vi "APU Page.vi"(8 "error in (no error)":errorcluster, 11 "Node Ptr":T1 format="%.0x") -> (0 "error out":errorcluster)   [LabVIEW 2015, in "Engine Simulation Toolkit System Explorer.lvlib"]
uses:
  Engine Simulation Toolkit System Explorer.lvlib
  <vilib>/NI Veristand/Custom Device API/Custom Device Item Ref.ctl
  Shared/Properties.vi
  <vilib>/NI Veristand/Custom Device API/Get Item Property (U16).vi
  <vilib>/NI Veristand/Custom Device API/Get Item Property (Double).vi
  <vilib>/NI Veristand/Custom Device API/Get Item Property (String).vi
  <vilib>/NI Veristand/Custom Device API/Get Item Property (Boolean).vi
  Shared/Constants and GUIDs.vi
  <vilib>/NI Veristand/Custom Device Tools/Custom Device Utility Library/NI VeriStand - Search for Item by Name.vi
  <vilib>/NI Veristand/Custom Device API/Set Item Property (Double).vi
  <vilib>/NI Veristand/Custom Device API/Set Item Property (Boolean).vi
  <vilib>/NI Veristand/Custom Device API/Custom Device API.lvlib
  Shared/Engine Simulation Toolkit Shared.lvlib
  <vilib>/NI Veristand/Custom Device Tools/Custom Device Utility Library/Custom Device Utility Library.lvlib
panel:
  in  "des speed":dbl caption="Start speed (RPM)"
  in  "Start angle (degrees)":dbl
  in  "des accel":dbl caption="Acceleration (RPM/sec)" min=0.0 format="%#_p"
  in  "Acceleration":bool
  out "Name in bitfile":string
  in  "Header":cluster{"Section Name":string}={"Section Name"="APU Settings"}
  in  "Description":string
  in  "Name":string
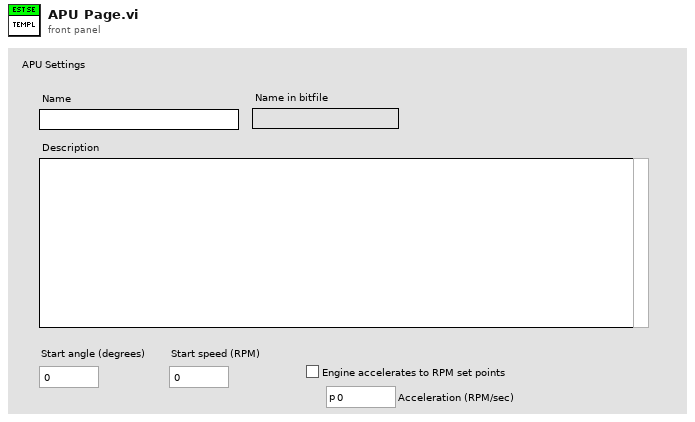
[diagram p1: front panel]
types:
  T1 = typedef "Custom Device API.lvlib/Custom Device Item Ref.ctl" = u64
  T2 = enum8{"Enabled", "Disabled", "Disabled and Grayed Out"}
  T3 = typedef "Engine Simulation Toolkit Shared.lvlib/Channel.ctl" = cluster{"Name":string, "Units":string, "Default":dbl, "Description":string}
  T4 = typedef "Custom Device API.lvlib/Custom Device Channel.ctl" = cluster{"Type":T5, "Units":string, "Default Value":dbl, "Faultable":bool, "Scalable":bool}
  T5 = typedef "Custom Device API.lvlib/Custom Device Channel Type.ctl" = enum16{"Input", "Output"}
  T6 = typedef "Custom Device API.lvlib/Custom Device Item Info.ctl" = cluster{"Name":string, "Is Channel":bool, "GUID":string, "Is Waveform":bool}
  T7 = typedef "Custom Device API.lvlib/Custom Device Commands.ctl" = enum16{"Default", "Item renamed", "Shutdown", "Dynamic button pressed"}
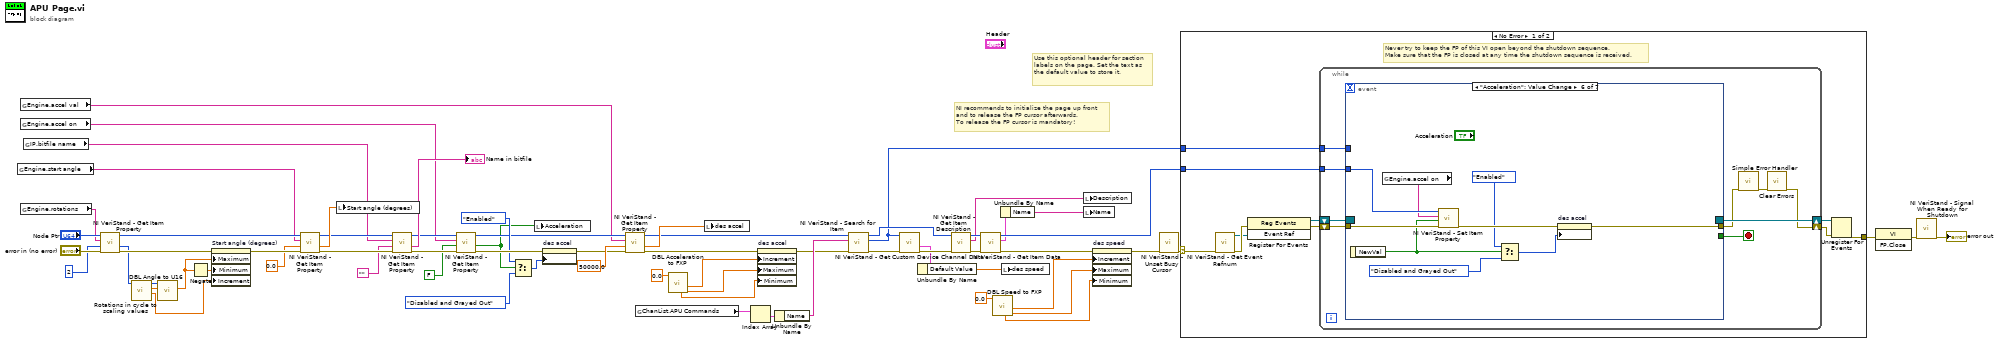
[diagram p0: block diagram]
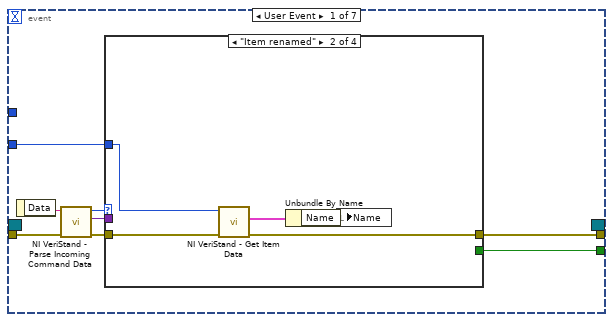
[diagram p2: hidden frame]
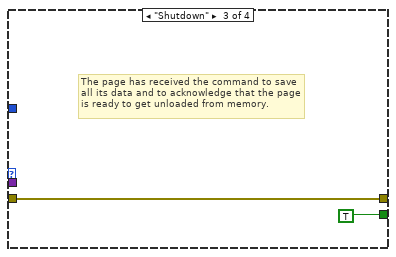
[diagram p4: hidden frame]
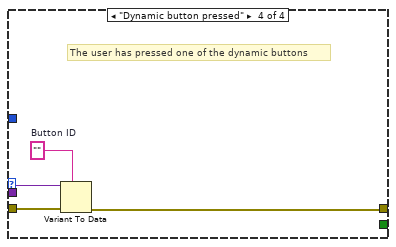
[diagram p5: hidden frame]
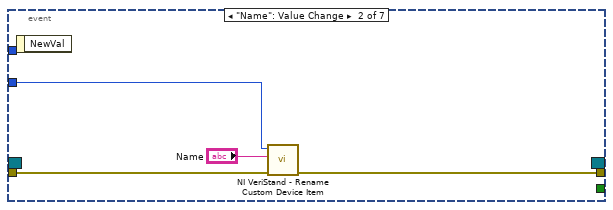
[diagram p6: hidden frame]
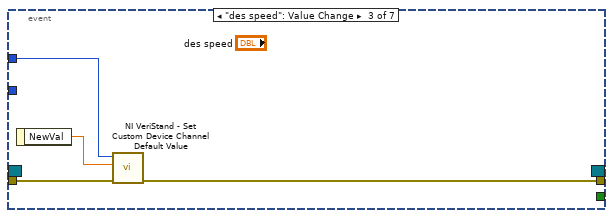
[diagram p7: hidden frame]
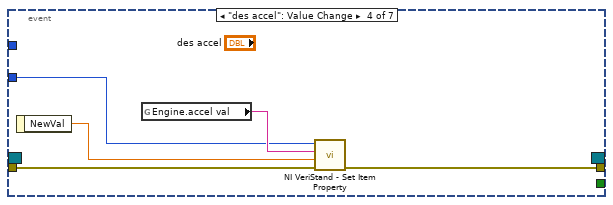
[diagram p8: hidden frame]
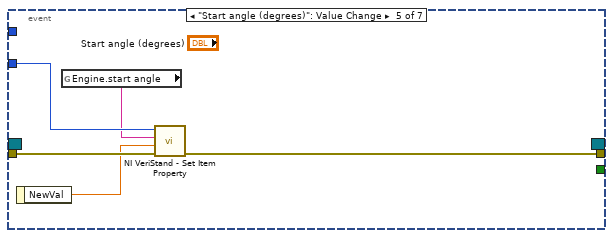
[diagram p9: hidden frame]
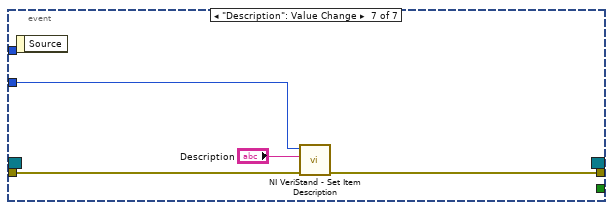
[diagram p10: hidden frame]
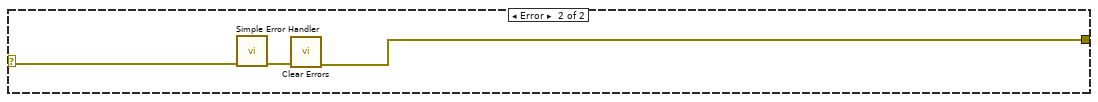
[diagram p11: hidden frame]
diagram:
  # "Use this optional header for section labels on the page. Set the text as the default value to store it."
  # "NI recommends to initialize the page up front\nand to release the FP cursor afterwards.\nTo release the FP cursor is mandatory!"
  n1 = global read "Properties.vi" "Engine.start angle"() -> (w50:string)
  n2 = global read "Properties.vi" "Engine.rotations"() -> (w54:string)
  n3 = global read "Properties.vi" "Engine.accel val"() -> (w34:string)
  n4 = global read "Properties.vi" "Engine.accel on"() -> (w40:string)
  n5 = global read "Properties.vi" "IP.bitfile name"() -> (w44:string)
  n6 = call-poly <vilib>:"NI VeriStand - Get Item Property.vi"("error in (no error)"="error in (no error)", "Default Value"=u16 2, "Property Name"=w54, "Item Ref in"="Node Ptr") -> ("error out"=w56:errorcluster, "Value"=w18:u16, "Item Ref out"=w51:T1)  [unwired: 4 in, 1 out]
  n7 = call "Rotations in cycle to scaling values.vi"("rotations in a cycle"=w18) -> ("degrees of one u16"=w14:dbl, "angle to u16 scale factor"=w16:dbl, "total angle span (degrees)"=w17:u16)  [unwired: 8 in]
  n8 = call "DBL Angle to U16.vi"("angle to u16 scale factor"=w16, "Desired angle (degrees)"=w17) -> ("Actual angle (degrees)"=w15:dbl)  [unwired: 8 in, 1 out]
  n9 = Negate(x=w15) -> (-x=w19:dbl)
  n10 = property on="Start angle (degrees)" class="DigNum (strict)"(error in=w56, "Maximum"=w15, "Minimum"=w19, "Increment"=w14) -> (error out=w49:errorcluster)  [unwired: 1 in, 1 out]
  n11 = call-poly <vilib>:"NI VeriStand - Get Item Property.vi"("error in (no error)"=w49, "Default Value"=0.0, "Property Name"=w50, "Item Ref in"=w51) -> ("error out"=w52:errorcluster, "Value"=w47:dbl, "Item Ref out"=w45:T1)  [unwired: 4 in, 1 out]
  n12 = local write "Start angle (degrees)"(w47) -> ()
  n13 = call-poly <vilib>:"NI VeriStand - Get Item Property.vi"("error in (no error)"=w52, "Default Value"="", "Property Name"=w44, "Item Ref in"=w45) -> ("error out"=w46:errorcluster, "Value"=→"Name in bitfile":string, "Item Ref out"=w41:T1)  [unwired: 4 in, 1 out]
  n14 = call-poly <vilib>:"NI VeriStand - Get Item Property.vi"("error in (no error)"=w46, "Default Value"=FALSE, "Property Name"=w40, "Item Ref in"=w41) -> ("error out"=w38:errorcluster, "Value"=w20:bool, "Item Ref out"=w35:T1)  [unwired: 4 in, 1 out]
  n15 = Select(t=T2."Enabled" ("Disabled"), s=w20, f=T2."Disabled and Grayed Out" ("Disabled")) -> (s? t:f=w33:T2)
  n16 = local write "Acceleration"(w20) -> ()
  n17 = property on="des accel" class="DigNum (strict)"(error in=w38, "DisabledEnum"=w33) -> (error out=w1:errorcluster)  [unwired: 1 in, 1 out]
  n18 = call-poly <vilib>:"NI VeriStand - Get Item Property.vi"("error in (no error)"=w1, "Default Value"=50000.0, "Property Name"=w34, "Item Ref in"=w35) -> ("error out"=w7:errorcluster, "Value"=w31:dbl, "Item Ref out"=w29:T1)  [unwired: 4 in, 1 out]
  n19 = global read "Constants and GUIDs.vi" "ChanList.APU Commands"() -> (w28:T3[])
  n20 = call "DBL Acceleration to FXP.vi"("Desired acceleration (RPM/sec)"=0.0) -> ("accel max"=w5:dbl, "accel resolution"=w6:dbl, "accel min"=w4:dbl)  [unwired: 6 in, 2 out]
  n21 = local write "des accel"(w31) -> ()
  n22 = Index Array(array=w28) -> (element=w27:T3)  [unwired: 1 in]
  n23 = property on="des accel" class="DigNum (strict)"(error in=w7, "Increment"=w6, "Maximum"=w5, "Minimum"=w4) -> (error out=w8:errorcluster)  [unwired: 1 in, 1 out]
  n24 = Unbundle By Name(w27) -> ("Name"=w26:string)
  n25 = call-poly <vilib>:"NI VeriStand - Search for Item.vi"("error in"=w8, "Item Name"=w26, "Section Ref in"=w29) -> ("error out"=w30:errorcluster, "Item Ref"=w21:T1, "Section Ref out"=w24:T1)  [unwired: 5 in, 1 out]
  n26 = call <vilib>:"NI VeriStand - Get Custom Device Channel Data.vi"("error in (no error)"=w30, "Channel Ref in"=w21) -> ("error out"=w25:errorcluster, "Channel"=w23:T4)  [unwired: 4 in, 4 out]
  n27 = Unbundle By Name(w23) -> ("Default Value"=w22:dbl)
  n28 = call <vilib>:"NI VeriStand - Get Item Description.vi"("error in (no error)"=w25, "Item Ref in"=w24) -> ("error out"=w59:errorcluster, "Description"=w60:string, "Item Ref out"=w61:T1)  [unwired: 7 out]
  n29 = call <vilib>:"NI VeriStand - Get Item Data.vi"("error in (no error)"=w59, "Item Ref in"=w61) -> ("error out"=w13:errorcluster, "Item Info"=w58:T6, "Item Ref out"=w62:T1)  [unwired: 7 out]
  n30 = call "DBL Speed to FXP.vi"("Desired speed (RPM)"=0.0) -> ("rpm max"=w10:dbl, "rpm resolution"=w11:dbl, "rpm min"=w9:dbl)  [unwired: 6 in, 2 out]
  n31 = Unbundle By Name(w58) -> ("Name"=w57:string)
  n32 = local write "des speed"(w22) -> ()
  n33 = local write "Description"(w60) -> ()
  n34 = local write "Name"(w57) -> ()
  n35 = property on="des speed" class="DigNum (strict)"(error in=w13, "Increment"=w11, "Maximum"=w10, "Minimum"=w9) -> (error out=w12:errorcluster)  [unwired: 1 in, 1 out]
  n36 = call <vilib>:"NI VeriStand - Unset Busy Cursor.vi"("error in (no error)"=w12) -> ("error out"=w64:errorcluster)  [unwired: 10 out]
  n37 = case shown="No Error" w64 {
    selector: w64 -> [w69 w140]
    tunnel: [w74 w138] -> w67
    tunnel: w62 -> [w70 _]
    tunnel: w21 -> [w68 _]
    frame No Error {
      # "Never try to keep the FP of this VI open beyond the shutdown sequence.\nMake sure that the FP is closed at any time the shutdown sequence is received."
      n38 = call <vilib>:"NI VeriStand - Get Event Refnum.vi"("error in (no error)"=w69) -> ("error out"=w77:errorcluster, "Event Ref"=w73:refnum<user-event>)  [unwired: 9 out]
      n39 = register-events(error in=w77, w73) -> (reference out=w71:refnum<event-registration>, error out=w72:errorcluster)  [unwired: 1 in]
      n40 = while {
        tunnel: w70 -> [w82]
        shift-right: [w79] -> w75
        shift-left: w72 -> [w85]
        shift-right: [w86] -> w76
        shift-left: w71 -> [w84]
        tunnel: w68 -> [w78]
        stop <- w83 stop-if-true
        n41 = event shown="[5] \"Acceleration\": Value Change" {
          selector: w84 -> [_ _ _ _ _ _ _]
          dyn-events: [_ _ _ _ _ _ _] -> w86
          timeout: _ -> [_ _ _ _ _ _ _]
          tunnel: w85 -> [w94 w110 w114 w119 w124 w133 w136]
          tunnel: [w90 _ _ _ _ _ _] -> w83
          tunnel: [w89 w109 w112 w118 w123 w125 w135] -> w81
          tunnel: w82 -> [w88 w108 _ w115 w122 w132 w137]
          tunnel: w78 -> [_ _ w113 _ _ _ _]
          event User Event {
            n42 = event-data() -> ("Data"=w93:string)  [unwired: 1 out]
            n43 = call <vilib>:"NI VeriStand - Parse Incoming Command Data.vi"("error in (no error)"=w94, "Incoming data"=w93) -> ("error out"=w92:errorcluster, "Outgoing data"=w87:variant, "Action"=w91:T7)  [unwired: 7 out]
            n44 = case shown="\"Item renamed\"" w91 {
              tunnel: w92 -> [w95 w100 w101 w106]
              tunnel: [_ _ TRUE _] -> w90
              tunnel: [w95 w97 w101 w103] -> w89
              tunnel: w88 -> [_ w99 _ _]
              tunnel: w87 -> [_ _ _ w105]
              frame "Default", Default {
              }
              frame "Item renamed" {
                n45 = call <vilib>:"NI VeriStand - Get Item Data.vi"("error in (no error)"=w100, "Item Ref in"=w99) -> ("error out"=w97:errorcluster, "Item Info"=w98:T6)  [unwired: 8 out]
                n46 = Unbundle By Name(w98) -> ("Name"=w96:string)
                n47 = local write "Name"(w96) -> ()
              }
              frame "Shutdown" {
                # "The page has received the command to save all its data and to acknowledge that the page is ready to get unloaded from memory."
              }
              frame "Dynamic button pressed" {
                w104 = ""  # Button ID
                # "The user has pressed one of the dynamic buttons"
                n48 = Variant To Data(error in=w106, type=w104, Variant=w105) -> (error out=w103:errorcluster)  [unwired: 1 out]
              }
            }
          }
          event "Name": Value Change {
            n49 = event-data() -> ()  [unwired: 2 out]
            n50 = call <vilib>:"NI VeriStand - Rename Custom Device Item.vi"("error in (no error)"=w110, "New Name"="Name", "Item Ref in"=w108) -> ("error out"=w109:errorcluster)  [unwired: 1 in, 7 out]
          }
          event "des speed": Value Change {
            n51 = event-data() -> ("NewVal"=w111:dbl)  [unwired: 1 out]
            n52 = call <vilib>:"NI VeriStand - Set Custom Device Channel Default Value.vi"("error in (no error)"=w114, "Default Value"=w111, "Channel Ref in"=w113) -> ("error out"=w112:errorcluster)  [unwired: 7 in, 1 out]
          }
          event "des accel": Value Change {
            n53 = event-data() -> ("NewVal"=w117:dbl)  [unwired: 1 out]
            n54 = global read "Properties.vi" "Engine.accel val"() -> (w116:string)
            n55 = call-poly <vilib>:"NI VeriStand - Set Item Property.vi"("error in (no error)"=w119, "Value"=w117, "Property Name"=w116, "Item Ref in"=w115) -> ("error out"=w118:errorcluster)  [unwired: 5 in, 2 out]
          }
          event "Start angle (degrees)": Value Change {
            n56 = event-data() -> ("NewVal"=w121:dbl)  [unwired: 1 out]
            n57 = global read "Properties.vi" "Engine.start angle"() -> (w120:string)
            n58 = call-poly <vilib>:"NI VeriStand - Set Item Property.vi"("error in (no error)"=w124, "Value"=w121, "Property Name"=w120, "Item Ref in"=w122) -> ("error out"=w123:errorcluster)  [unwired: 5 in, 2 out]
          }
          event "Acceleration": Value Change {
            n59 = event-data() -> ("NewVal"=w129:bool)  [unwired: 1 out]
            n60 = global read "Properties.vi" "Engine.accel on"() -> (w131:string)
            n61 = call-poly <vilib>:"NI VeriStand - Set Item Property.vi"("error in (no error)"=w133, "Value"=w129, "Property Name"=w131, "Item Ref in"=w132) -> ("error out"=w130:errorcluster)  [unwired: 5 in, 2 out]
            n62 = Select(t=T2."Enabled" ("Disabled"), s=w129, f=T2."Disabled and Grayed Out" ("Disabled")) -> (s? t:f=w127:T2)
            n63 = property on="des accel" class="DigNum (strict)"(error in=w130, "DisabledEnum"=w127) -> (error out=w125:errorcluster)  [unwired: 1 in, 1 out]
          }
          event "Description": Value Change {
            n64 = event-data() -> ()  [unwired: 2 out]
            n65 = call <vilib>:"NI VeriStand - Set Item Description.vi"("error in (no error)"=w136, "Description"="Description", "Item Ref in"=w137) -> ("error out"=w135:errorcluster)  [unwired: 8 out]
          }
        }
        n66 = call <vilib>:"Simple Error Handler.vi"("error in (no error)"=w81) -> ("error out"=w80:errorcluster)  [unwired: 1 in, 7 out]
        n67 = call <vilib>:"Clear Errors.vi"("error in (no error)"=w80) -> ("error out"=w79:errorcluster)  [unwired: 1 in, 5 out]
      }
      n68 = Unregister For Events(event registration refnum=w76, error in=w75) -> (error out=w74:errorcluster)
    }
    frame Error {
      n69 = call <vilib>:"Simple Error Handler.vi"("error in (no error)"=w140) -> ("error out"=w139:errorcluster)  [unwired: 1 in, 7 out]
      n70 = call <vilib>:"Clear Errors.vi"("error in (no error)"=w139) -> ("error out"=w138:errorcluster)  [unwired: 1 in, 5 out]
    }
  }
  n71 = invoke class="VI" method="FP.Close"(error in=w67) -> (error out=w66:errorcluster)  [unwired: 2 in, 2 out]
  n72 = call <vilib>:"NI VeriStand - Signal When Ready for Shutdown.vi"("error in (no error)"=w66) -> ("error out"=→"error out":errorcluster)  [unwired: 10 out]
